vi "Create Bitfile Dependency.vi"(8 "error in (no error)":errorcluster, 10 "Bitfile Path":path, 11 "Item Ref in":T1 format="%.0x") -> (0 "error out":errorcluster, 3 "Device Ref out":T1 format="%.0x")   [LabVIEW 2015, in "Diagnostics Addon Shared.lvlib"]
uses:
  Diagnostics Addon Shared.lvlib
  <vilib>/NI Veristand/Custom Device API/Custom Device Item Ref.ctl
  <vilib>/NI Veristand/Custom Device API/Custom Device File Dependency.ctl
  <vilib>/NI Veristand/Custom Device API/Path Specification.ctl
  <vilib>/NI Veristand/Custom Device API/Path Type.ctl
  <vilib>/NI Veristand/Custom Device API/Custom Device Supported Target.ctl
  GUID Lookup.vi
  <vilib>/NI Veristand/Custom Device API/Set Item Property (Path).vi
  <vilib>/NI Veristand/Custom Device API/Custom Device API.lvlib
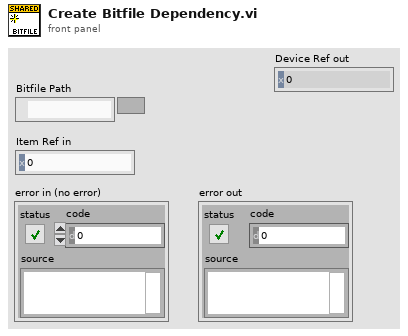
[diagram p1: front panel]
types:
  T1 = typedef "Custom Device API.lvlib/Custom Device Item Ref.ctl" = u64
  T2 = typedef "Custom Device API.lvlib/Custom Device File Dependency.ctl" = cluster{"Source":T3, "RT Destination":path, "ForceDownload?":bool, "SupportedTarget":T5, "Version":string}
  T3 = typedef "Custom Device API.lvlib/Path Specification.ctl" = cluster{"Path":path, "Type":T4}
  T4 = typedef "Custom Device API.lvlib/Path Type.ctl" = enum16{"Absolute", "To Base", "To Common Data Dir", "To Application Data Dir"}
  T5 = typedef "Custom Device API.lvlib/Custom Device Supported Target.ctl" = enum16{"All", "PharLap", "VxWorks", "Windows", "Linux_32_ARM", "Linux_x64", "PharLap & Windows", "PharLap & VxWorks", "VxWorks & Windows"}
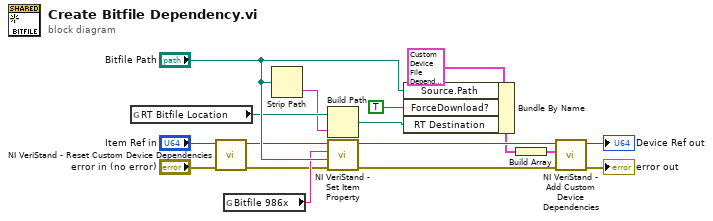
[diagram p0: block diagram]
diagram:
  n1 = global read "GUID Lookup.vi" "RT Bitfile Location"() -> (w13:path)
  n2 = call <vilib>:"NI VeriStand - Reset Custom Device Dependencies.vi"("error in (no error)"="error in (no error)", "Device Ref in"="Item Ref in") -> ("error out"=w8:errorcluster, "Device Ref out"=w11:T1)  [unwired: 8 in]
  n3 = global read "GUID Lookup.vi" "Bitfile 986x"() -> (w12:string)
  n4 = Strip Path(path="Bitfile Path") -> (name=w6:string)  [unwired: 1 out]
  n5 = Build Path(base path=w13, name or relative path=w6) -> (appended path=w7:path)
  n6 = call-poly <vilib>:"NI VeriStand - Set Item Property.vi"("error in (no error)"=w8, "Value"="Bitfile Path", "Property Name"=w12, "Item Ref in"=w11) -> ("error out"=w9:errorcluster, "Item Ref out"=w10:T1)  [unwired: 5 in, 1 out]
  n7 = Bundle By Name(cluster=T2 {"Source"={"Path"=path "", "Type"=enum."Absolute"}, "RT Destination"=path "", "ForceDownload?"=FALSE, "SupportedTarget"=enum."PharLap", "Version"=""} ("Dependency"), "Source.Path"="Bitfile Path", "ForceDownload?"=TRUE, "RT Destination"=w7) -> (w3:T2)
  n8 = Build Array(w3) -> (w4:T2[])
  n9 = call <vilib>:"NI VeriStand - Add Custom Device Dependencies.vi"("error in (no error)"=w9, "Dependencies"=w4, "Device Ref in"=w10) -> ("error out"=→"error out":errorcluster, "Device Ref out"=→"Device Ref out":T1)  [unwired: 7 in]
